vi "ConvertDocxToMDUsingWritage.vi"() -> ()   [LabVIEW 2018]
uses:
  <vilib>/regexp/Match Regular Expression.xnode
panel:
  out "String 2":string
  out "FiguresCaptionTexts":string[](array[string])
  out "FiguresNumbers":string[](array[string])
  out "String":string
  in  "file path (use dialog)":path=path "C:/Users/jgsaenz/gitRepos/HMIComputers_documentation/00 Structure/LSST_HMI_SoftwareDocumentation_0_Structure.md"
  # "This VI mus be used after saving the docx file as md using the writage tool"
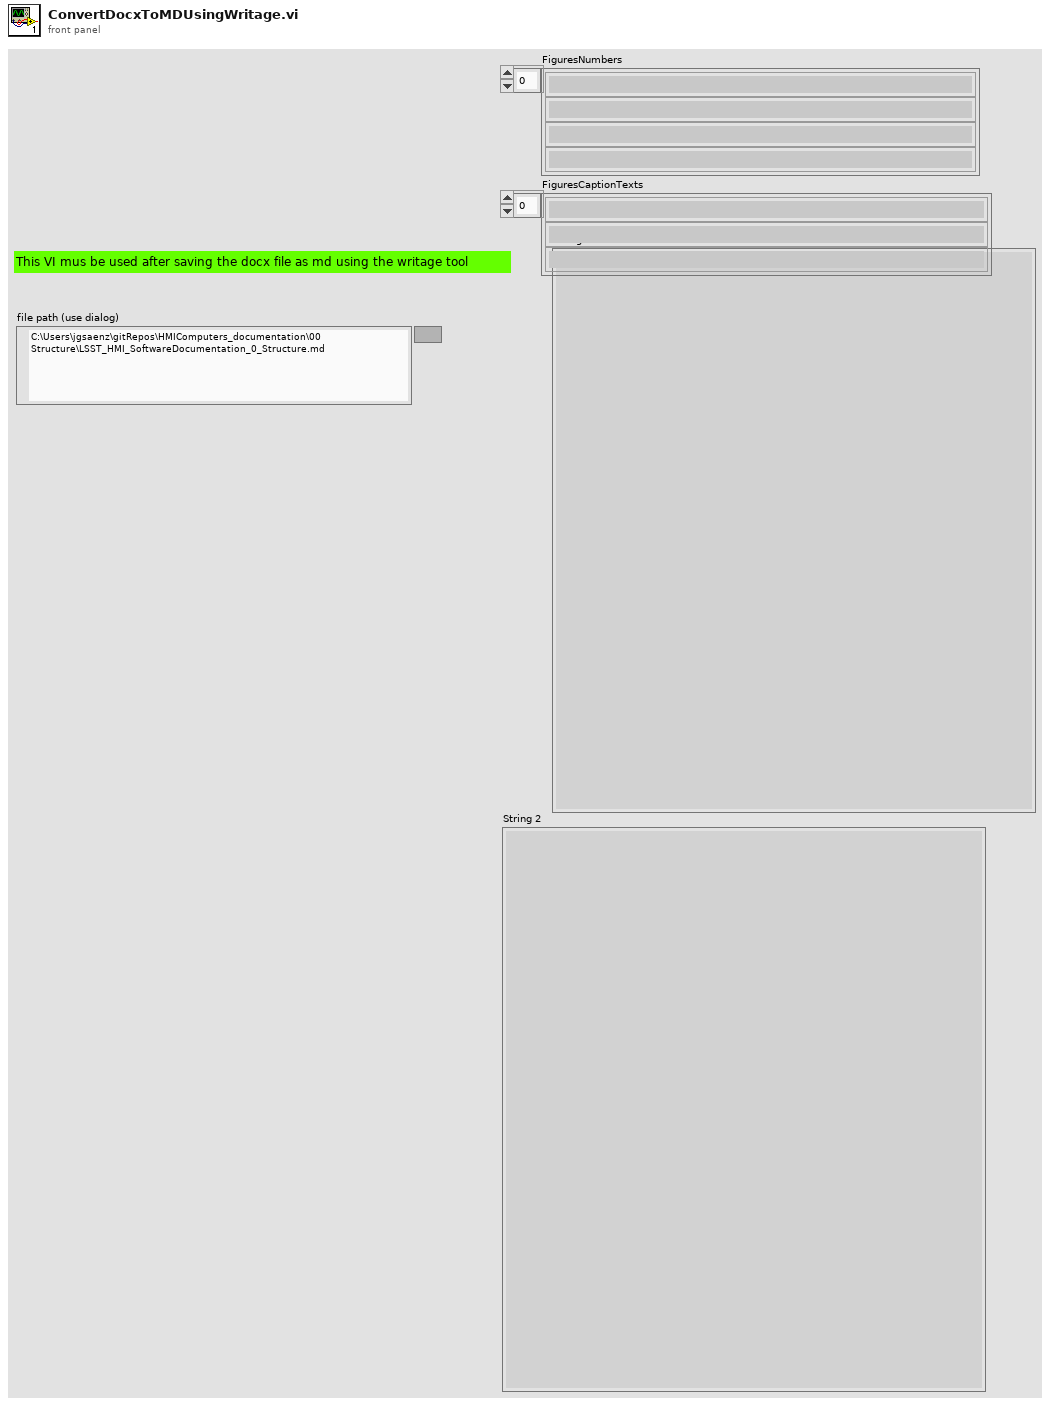
[diagram p1: front panel]
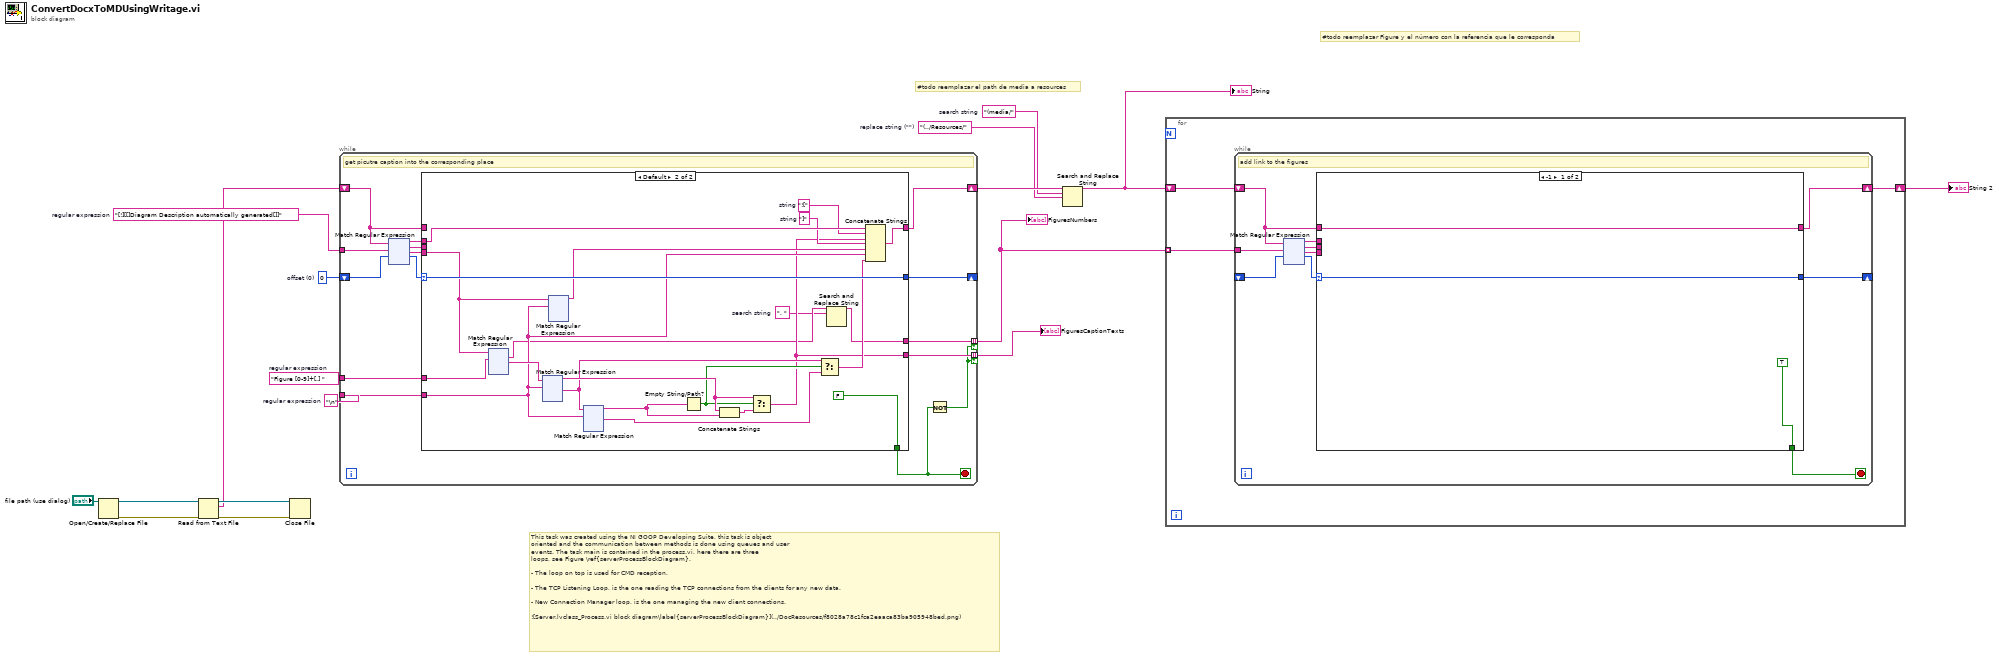
[diagram p0: block diagram]
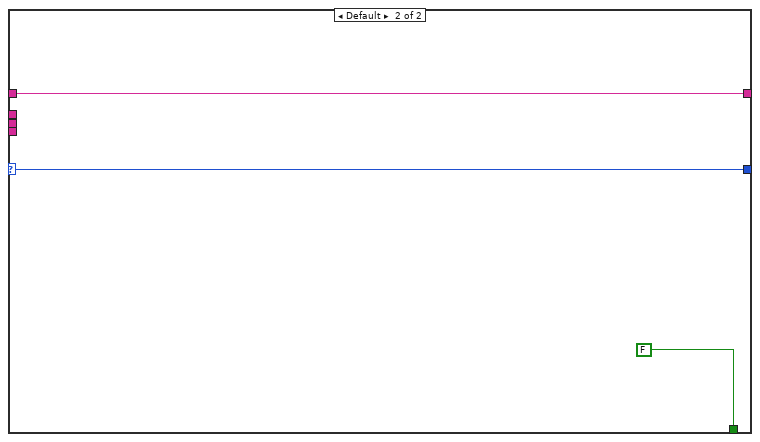
[diagram p2: hidden frame]
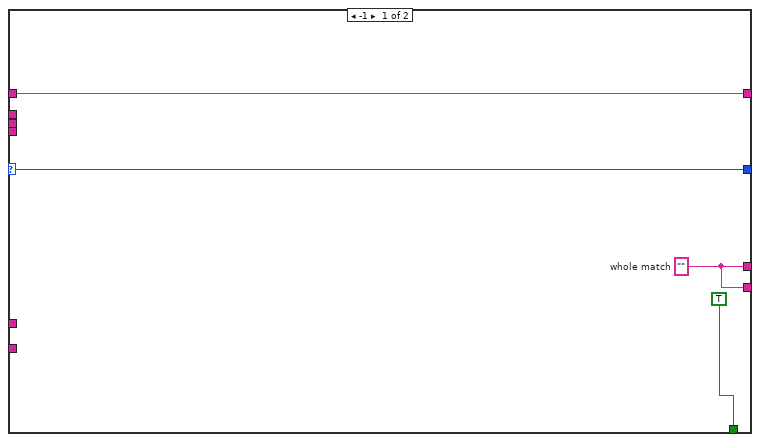
[diagram p3: hidden frame]
diagram:
  w5 = "(../Resources/"  # replace string ("")
  w6 = "(media/"  # search string
  w8 = 0  # offset (0)
  w9 = "\n"  # regular expression
  w10 = "Figure [0-9]+[.] "  # regular expression
  w11 = "[!][[]Diagram Description automatically generated[]]"  # regular expression
  # "#todo reemplazar el path de media a resources"
  # "#todo reemplazar Figure y el número con la referencia que le corresponda"
  # "This task was created using the NI GOOP Developing Suite, this task is object\noriented and the communication between methods is done using queues and user\nevents. The task main is contained in the process.vi, here there are three\nloops, see Figure \\ref{serverProcessBlockDiagram}.\n\n- The loop on top is used for CMD reception.\n\n- The TCP Listening Loop, is the one reading the TCP connections from the clients for any new data.\n\n- New Connection Manager loop, is the one managing the new client connections.\n\n![Server.lvclass_Process.vi block diagram\\label{serverProcessBlockDiagram}](../DocResources/f8028a78c1fca2eaaca83ba905948bed.png)"
  n1 = Open/Create/Replace File(file path (use dialog)="file path (use dialog)") -> (refnum out=w16:refnum<file>, error out=w17:errorcluster)  [unwired: 5 in, 1 out]
  n2 = Read from Text File(file (use dialog)=w16, error in=w17) -> (refnum out=w14:refnum<file>, text=w12:string, error out=w15:errorcluster)  [unwired: 2 in, 1 out]
  n3 = Close File(refnum=w14, error in=w15) -> ()  [unwired: 2 out]
  n4 = while {
    tunnel: w11 -> [w32]
    tunnel: w10 -> [w31]
    tunnel: w9 -> [w29]
    shift-right: [w26] -> _
    shift-left: w8 -> [w28]
    shift-right: [w24] -> w7
    shift-left: w12 -> [w25]
    tunnel: [w21] -> w1 mode=indexing if=w18
    tunnel: [w20] -> w4 mode=indexing if=w18
    stop <- w19 stop-if-true
    # "get picutre caption into the corresponding place"
    n5 = xnode "Match Regular Expression"("input string"=w25, "regular expression"=w32, "offset (0)"=w28) -> ("before match"=w22:string, "whole match"=w23:string, "after match"=w30:string, "offset past match"=w27:i32)  [unwired: 3 in, 1 out]
    n6 = case shown="Default" w27 {
      selector: w27 -> [w36 w53]
      tunnel: w31 -> [_ w58]
      tunnel: w30 -> [_ w47]
      tunnel: w29 -> [_ w45]
      tunnel: [w36 w53] -> w26
      tunnel: w25 -> [w35 _]
      tunnel: [w35 w51] -> w24
      tunnel: w23 -> [_ _]
      tunnel: w22 -> [_ w52]
      tunnel: [TRUE FALSE] -> w19
      tunnel: [w33 w38] -> w21
      tunnel: [w33 w40] -> w20
      frame -1 {
        w33 = ""  # whole match
      }
      frame Default {
        w37 = ". "  # search string
        w49 = "]"  # string
        w50 = "!["  # string
        n7 = xnode "Match Regular Expression"("input string"=w47, "regular expression"=w58) -> ("whole match"=w39:string, "after match"=w57:string)  [unwired: 4 in, 3 out]
        n8 = xnode "Match Regular Expression"("input string"=w57, "regular expression"=w45) -> ("before match"=w56:string, "after match"=w43:string)  [unwired: 4 in, 3 out]
        n9 = xnode "Match Regular Expression"("input string"=w47, "regular expression"=w45) -> ("before match"=w46:string)  [unwired: 4 in, 4 out]
        n10 = xnode "Match Regular Expression"("input string"=w43, "regular expression"=w45) -> ("before match"=w54:string, "after match"=w42:string)  [unwired: 4 in, 3 out]
        n11 = Empty String/Path?(string/path=w54) -> (empty?=w44:bool)
        n12 = Concatenate Strings(w56, w54) -> (w55:string)
        n13 = Select(t=w56, s=w44, f=w55) -> (s? t:f=w40:string)
        n14 = Select(t=w43, s=w44, f=w42) -> (s? t:f=w41:string)
        n15 = Search and Replace String(input string=w39, search string=w37) -> (result string=w38:string)  [unwired: 6 in, 3 out]
        n16 = Concatenate Strings(w52, w50, w40, w49, w46, w45, w41) -> (w51:string)
      }
    }
    n17 = Not(x=w19) -> (.not. x?=w18:bool)
  }
  "FiguresNumbers" <- w1
  "FiguresCaptionTexts" <- w4
  n18 = Search and Replace String(input string=w7, search string=w6, replace string=w5) -> (result string=w3:string)  [unwired: 5 in, 3 out]
  "String" <- w3
  n19 = for {
    tunnel: w1 -> [w629] mode=indexing
    shift-right: [w630] -> w2
    shift-left: w3 -> [w631]
    n20 = while {
      tunnel: w629 -> [w641]
      shift-right: [w637] -> _
      shift-left: _ -> [w639]
      shift-right: [w635] -> w630
      shift-left: w631 -> [w636]
      stop <- w632 stop-if-true
      # "add link to the figures"
      n21 = xnode "Match Regular Expression"("input string"=w636, "regular expression"=w641, "offset (0)"=w639) -> ("before match"=w633:string, "whole match"=w634:string, "after match"=w640:string, "offset past match"=w638:i32)  [unwired: 3 in, 1 out]
      n22 = case shown="-1" w638 {
        selector: w638 -> [w644 w646]
        tunnel: w640 -> [_ _]
        tunnel: [w644 w646] -> w637
        tunnel: w636 -> [w643 w645]
        tunnel: [w643 w645] -> w635
        tunnel: w634 -> [_ _]
        tunnel: w633 -> [_ _]
        tunnel: [TRUE FALSE] -> w632
        frame -1 {
        }
        frame Default {
        }
      }
    }
  }
  "String 2" <- w2
